vi "ATF-Pump-Seq AO  Executer.vi"(8 "error in":errorcluster) -> (0 "error IO":errorcluster)   [LabVIEW 2022 SP3]
uses:
  <vilib>/Platform/TimedLoop/XDataNode/timing_clust.ctl
  <vilib>/Platform/TimedLoop/XDataNode/nitl_modes.ctl
  <vilib>/Platform/TimedLoop/XDataNode/wakeup.ctl
  e3473751-051d-4c88-8500-c7ef790b628c.vi
  <vilib>/platform/TimedLoop/XDataNode/XDataNode.xnode
  <vilib>/Platform/TimedLoop/XDataNode/XDNodeRunTimeDep.lvlib
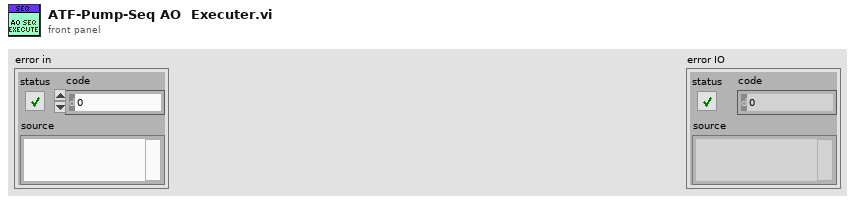
[diagram p1: front panel]
types:
  T1 = cluster{"Value":dbl[], "Name":string[], "SEQ":string[], "index":i32}
  T2 = typedef "XDNodeRunTimeDep.lvlib/timing_clust.ctl" = cluster{"Expected End [f-1]":u64, "Actual End [f-1]":u64, "Finished Late? [f-1]":bool, "Expected End [i-1]":u64, "Actual End [i-1]":u64, "Finished Late? [i-1]":bool, "Expected Start [i]":u64, "Actual Start [i]":u64, "Expected Start [f]":u64, "Actual Start [f]":u64, "Source Name":string, "Structure Name":string, "Period":i64, "Deadline":i64, "Offset":i64, "Start":i64, "Priority":i32, "Timeout":i32, "Mode":T3, "Wakeup Reason":T4, "Error":errorcluster, "Source Type":string, "Secondary Source Type":string, "Global End Time":u64, "Global Start Time":u64, "Frame Duration":u64, "Iteration Duration":u64, "Assigned CPU":i32, "I/O Scan Engine Mode":u32}
  T3 = typedef "XDNodeRunTimeDep.lvlib/nitl_modes.ctl" = enum32{"No Change", "Process missed periods, maintain original phase", "Discard missed periods, maintain original phase", "Process missed periods, ignore original phase", "Discard missed periods, ignore original phase"}
  T4 = typedef "XDNodeRunTimeDep.lvlib/wakeup.ctl" = enum32{"Normal", "Aborted", "Asynchronous wakeup", "Timing source error", "Timed loop error", "Timeout"}
  T5 = enum16{"Init", "Read", "Write 'All'", "Write 'n'", "Write Safe Value", "Write Start Time", "Read 1"}
  T6 = cluster{"Start DAQ":bool, "Stop DAQ":bool, "RT Stop":bool, "RT Exit":bool, "Start Seq":bool}
  T7 = cluster{"Manual HOLD":bool, "Automatic Hold AI":bool, "Abort":bool, "Automatic Hold DI":bool}
  T8 = cluster{cluster{"Sr. No.":string, "Time CDT":string, "Component ID":string, "Data Type":string, "Condition":string, "Range/Position":string, "No of Samples for Pass":string, "Event Duration":string, "Continuous /Cumulative":string, "Expected Delay":string, "Failure case Seq":string, "Current Sequence":string}[]}[]
  T9 = cluster{cluster{"Sr. No.":string, "Time CDT":string, "Component ID":string, "Data Type":string, "Condition":string, "Range/Position":string, "No of Samples for Pass":string, "Event Duration":string, "Continuous /Cumulative":string, "Expected Delay":string, "Failure case Seq":string, "Current Sequence":string}[]}
  T10 = cluster{"Sr. No.":string, "Time CDT":string, "Component ID":string, "Data Type":string, "Condition":string, "Range/Position":string, "No of Samples for Pass":string, "Event Duration":string, "Continuous /Cumulative":string, "Expected Delay":string, "Failure case Seq":string, "Current Sequence":string}[]
  T11 = cluster{"Sr. No.":string, "Time CDT":string, "Component ID":string, "Data Type":string, "Condition":string, "Range/Position":string, "No of Samples for Pass":string, "Event Duration":string, "Continuous /Cumulative":string, "Expected Delay":string, "Failure case Seq":string, "Current Sequence":string}
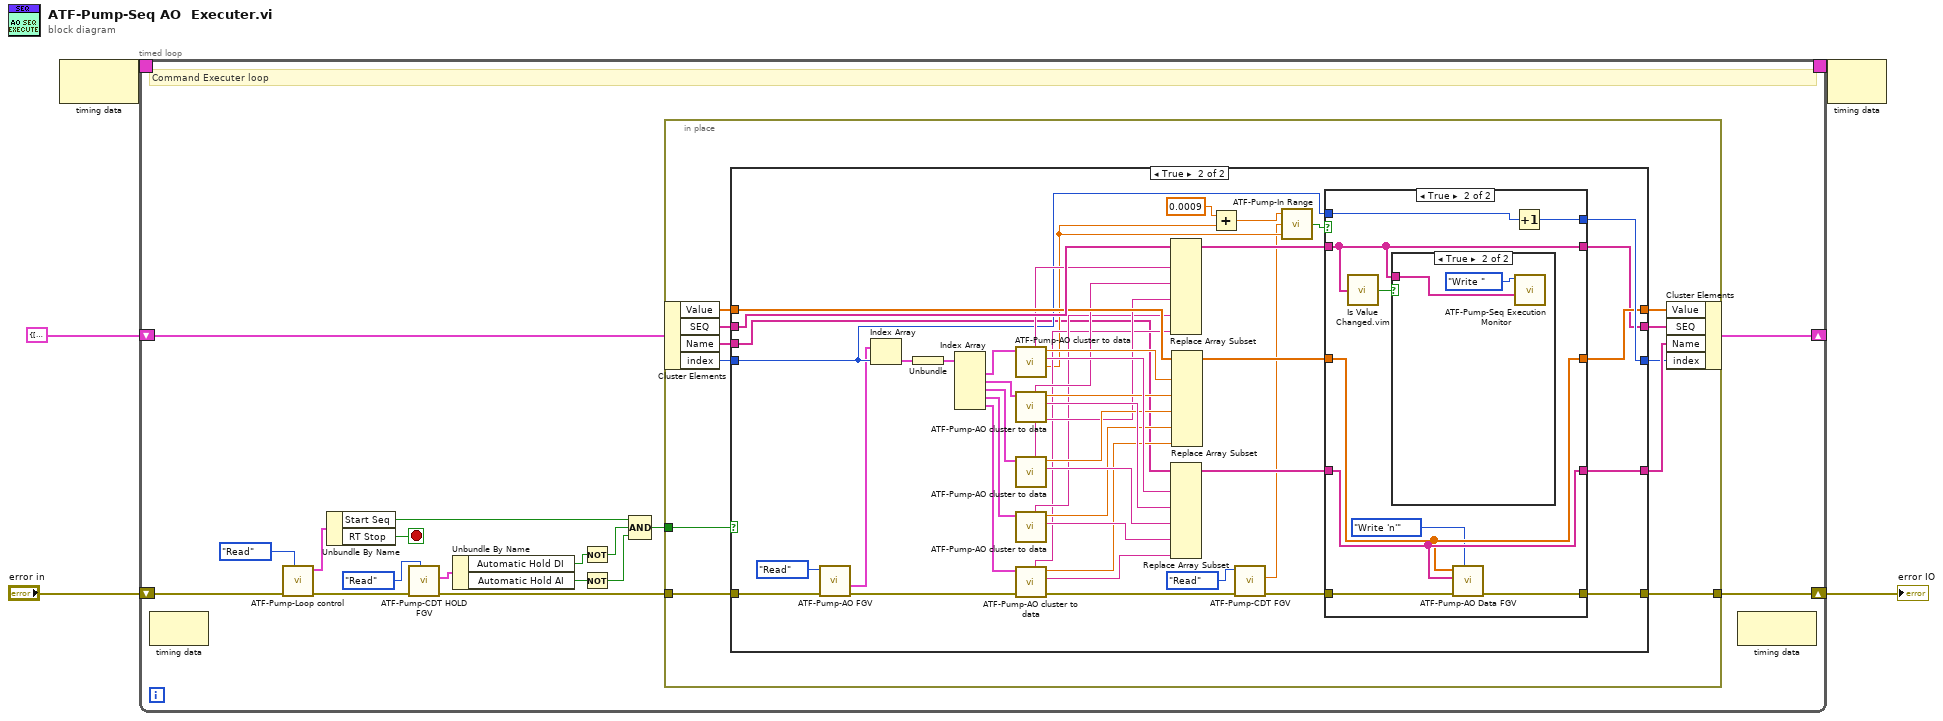
[diagram p0: block diagram]
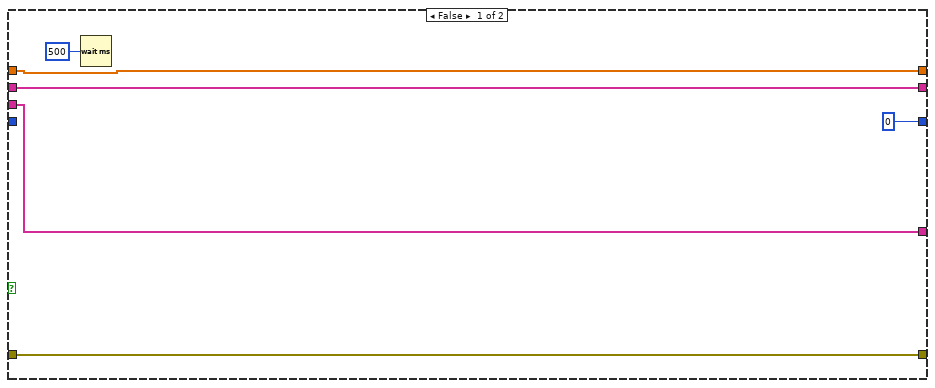
[diagram p2: hidden frame]
diagram:
  n1 = node-c288() -> (w5:T2)  [unwired: 1 in]
  n2 = timed-loop {
    shift-right: [w18] -> w1
    shift-left: "error in" -> [w21]
    timing: w5 -> [_]
    timing-out: [_] -> w4
    shift-right: [w6] -> _
    shift-left: T1 {"Value"=[0.0, 0.0, 0.0, 0.0, 0.0], "Name"=["", "", "", "", ""], "SEQ"=["", "", "", "", ""], "index"=0} -> [w7]
    stop <- w22 stop-if-true
    # "Command Executer loop"
    n3 = node-c288() -> ()  [unwired: 1 in, 1 out]
    n4 = call "ATF-Pump-Loop control.vi"("Action"=enum16{"Init", "Write", "Read"}."Read", "error in (no error)"=w21) -> ("error Out"=w10:errorcluster, "Loop Control out"=w19:T6)  [unwired: 8 in]
    n5 = Unbundle By Name(w19) -> ("Start Seq"=w8:bool, "RT Stop"=w22:bool)
    n6 = call "ATF-Pump-CDT HOLD FGV.vi"("Write/Read"=enum16{"Write", "Read"}."Read", "error in (no error)"=w10) -> ("error Out"=w9:errorcluster, "HOLD and Abort Out"=w14:T7)  [unwired: 6 in]
    n7 = Unbundle By Name(w14) -> ("Automatic Hold DI"=w12:bool, "Automatic Hold AI"=w13:bool)
    n8 = Not(x=w12) -> (.not. x?=w11:bool)
    n9 = Not(x=w13) -> (.not. x?=w16:bool)
    n10 = Compound Arithmetic op=AND(w8, w11, w16) -> (w15:bool)
    n11 = in-place {
      in-place-border: [w33] -> w18
      in-place-border: w15 -> [w32]
      in-place-border: w9 -> [w31]
      n12 = in-place-cluster #1(w7) -> ("Value"=w30:dbl[], "SEQ"=w29:string[], "Name"=w28:string[], "index"=w27:i32)
      n13 = case shown="True" w32 {
        tunnel: w31 -> [w39 w42]
        tunnel: [w39 w84] -> w33
        tunnel: w29 -> [w35 w83]
        tunnel: w30 -> [w37 w82]
        tunnel: [w37 w47] -> w23
        tunnel: [w34 w44] -> w25
        tunnel: [w35 w45] -> w26
        tunnel: w27 -> [_ w48]
        tunnel: [0 ("index") w49] -> w24
        tunnel: w28 -> [w34 w46]
        frame False {
          n14 = Wait (ms)(milliseconds to wait=u32 500) -> ()  [unwired: 1 out]
        }
        frame True {
          n15 = call "ATF-Pump-AO FGV.vi"("error in"=w42, "Enum"=enum16{"Read", "Write "}."Read") -> ("error out"=w41:errorcluster, "AO Seq  OUT"=w40:T8)  [unwired: 8 in]
          n16 = Index Array(array=w40, index=w48) -> (element=w79:T9)
          n17 = Unbundle(w79) -> (w78:T10)
          n18 = Index Array(array=w78) -> (element #1=w55:T11, element #2=w77:T11, element #3=w76:T11, element #4=w75:T11, element #5=w74:T11)  [unwired: 5 in]
          n19 = call "ATF-Pump-AO cluster to data.vi"("output cluster"=w55) -> ("Numeric"=w53:dbl, "Component ID"=w72:string, "Value"=w67:dbl, "concatenated string"=w60:string)  [unwired: 7 in]
          n20 = call "ATF-Pump-AO cluster to data.vi"("output cluster"=w77) -> ("Component ID"=w71:string, "Value"=w66:dbl, "concatenated string"=w59:string)  [unwired: 7 in, 1 out]
          n21 = call "ATF-Pump-AO cluster to data.vi"("output cluster"=w76) -> ("Component ID"=w70:string, "Value"=w65:dbl, "concatenated string"=w58:string)  [unwired: 7 in, 1 out]
          n22 = call "ATF-Pump-AO cluster to data.vi"("output cluster"=w75) -> ("Component ID"=w69:string, "Value"=w64:dbl, "concatenated string"=w57:string)  [unwired: 7 in, 1 out]
          n23 = call "ATF-Pump-AO cluster to data.vi"("output cluster"=w74) -> ("Component ID"=w68:string, "Value"=w63:dbl, "concatenated string"=w56:string)  [unwired: 7 in, 1 out]
          n24 = Replace Array Subset(array=w83, new element #1=w60, new element #2=w59, new element #3=w58, new element #4=w57, new element #5=w56) -> (w81:string[])  [unwired: 5 in]
          n25 = Replace Array Subset(array=w46, new element #1=w72, new element #2=w71, new element #3=w70, new element #4=w69, new element #5=w68) -> (w80:string[])  [unwired: 5 in]
          n26 = Replace Array Subset(array=w82, new element #1=w67, new element #2=w66, new element #3=w65, new element #4=w64, new element #5=w63) -> (w62:dbl[])  [unwired: 5 in]
          n27 = Add(x=0.0009, y=w53) -> (x+y=w54:dbl)
          n28 = call "ATF-Pump-CDT FGV.vi"("error in (no error)"=w41, "Write/Read"=enum16{"Write", "Read"}."Read") -> ("error Out"=w61:errorcluster, "CDT Out"=w51:dbl)  [unwired: 8 in]
          n29 = call "ATF-Pump-In Range.vi"("Min"=w53, "X"=w51, "Max"=w54) -> ("In Range"=w50:bool)  [unwired: 2 in]
          n30 = case shown="True" w50 {
            tunnel: w61 -> [w89 w93]
            tunnel: [w89 w94] -> w84
            tunnel: w62 -> [w88 w91]
            tunnel: w80 -> [w85 w92]
            tunnel: w81 -> [w86 w95]
            tunnel: [w88 w91] -> w47
            tunnel: [w87 w96] -> w49
            tunnel: w48 -> [w87 w97]
            tunnel: [w86 w95] -> w45
            tunnel: [w85 w92] -> w44
            frame False {
            }
            frame True {
              n31 = call "Is Value Changed.vim"("value"=w95) -> ("changed or first call?"=w98:bool)
              n32 = case shown="True" w98 {
                tunnel: w95 -> [_ w100]
                frame False {
                }
                frame True {
                  n33 = call "ATF-Pump-Seq Execution Monitor.vi"("Seq Monitor"=w100, "Enum"=enum16{"Read", "Write "}."Write ") -> ()  [unwired: 8 in, 2 out]
                }
              }
              n34 = call "ATF-Pump-AO Data FGV.vi"("Option"=T5."Write 'n'", "error in (no error)"=w93, "AO Channel Names"=w92, "AO Values In"=w91) -> ("error out"=w94:errorcluster)  [unwired: 3 in, 4 out]
              n35 = Increment(x=w97) -> (x+1=w96:i32)
            }
          }
        }
      }
      n36 = in-place-cluster #1("Value"=w23, "SEQ"=w26, "Name"=w25, "index"=w24) -> (w6:T1)
    }
    n37 = node-c288() -> ()  [unwired: 1 in, 1 out]
  }
  "error IO" <- w1
  n38 = node-c288(w4) -> ()  [unwired: 1 out]
